vi "Pipe Var Intf - Read Variable - Double.vi"(8 "error in (no error)":errorcluster, 9 "max dims (0: scalar)":i32, 10 "variable name":string, 11 "GOLPI ref. in":T1={"pipe handle"={"lv_proc.dll file path"=path "", "process instance handle"=[], "debug mode"=FALSE, "debug data"=[]}, "fast read timeout [ms]"=500, "fast read settle time [ms]"=10, "fast read to multiple [ms]"=1, "max elements per input line"=100, "slow read timeout [ms]"=5000, "stdin double format specifier"="%_16e", "max elements per stdout output column"=100, "console mode bitstream"=FALSE, "bitstream first read timeout [ms]"=1000, "bitstream read timeout [ms]"=50, "struct transfer possible"=FALSE, "matlab mode"=FALSE, "var pipe write timeout [ms]"=5000, "variable pipe mode"=FALSE, "variable pipe buffer size [Bytes]"=10000000, "variable pipe block size [Bytes]"=1000000} {"variable pipe block size [Bytes]" format="%.0p"; "variable pipe buffer size [Bytes]" format="%.0p"}) -> (0 "error out":errorcluster, 2 "data out":dbl[][](array[numeric]), 3 "GOLPI ref. out":T1={"pipe handle"={"lv_proc.dll file path"=path "", "process instance handle"=[], "debug mode"=FALSE, "debug data"=[]}, "fast read timeout [ms]"=500, "fast read settle time [ms]"=10, "fast read to multiple [ms]"=1, "max elements per input line"=100, "slow read timeout [ms]"=5000, "stdin double format specifier"="", "max elements per stdout output column"=100, "console mode bitstream"=FALSE, "bitstream first read timeout [ms]"=1000, "bitstream read timeout [ms]"=50, "struct transfer possible"=FALSE, "matlab mode"=FALSE, "var pipe write timeout [ms]"=5000, "variable pipe mode"=FALSE, "variable pipe buffer size [Bytes]"=10000000, "variable pipe block size [Bytes]"=1000000} {"variable pipe block size [Bytes]" format="%.0p"; "variable pipe buffer size [Bytes]" format="%.0p"})   [LabVIEW 2020, in "GOLPI library.lvlib"]
doc: "Read matrix from Octave using pipe variable interface. In case of compatible non-doubles, casts to double. max dims defines maximum expected dimensions count."
uses:
  GOLPI library.lvlib
  Public/GOLPI reference Type Def.ctl
  LV Process source distribution/Pipe Handle.ctl
  <vilib>/Utility/error.llb/Error Cluster From Error Code.vi
  <vilib>/ErrorRing/Error Ring.xnode
  LV Process source distribution/LV Process library.lvlib
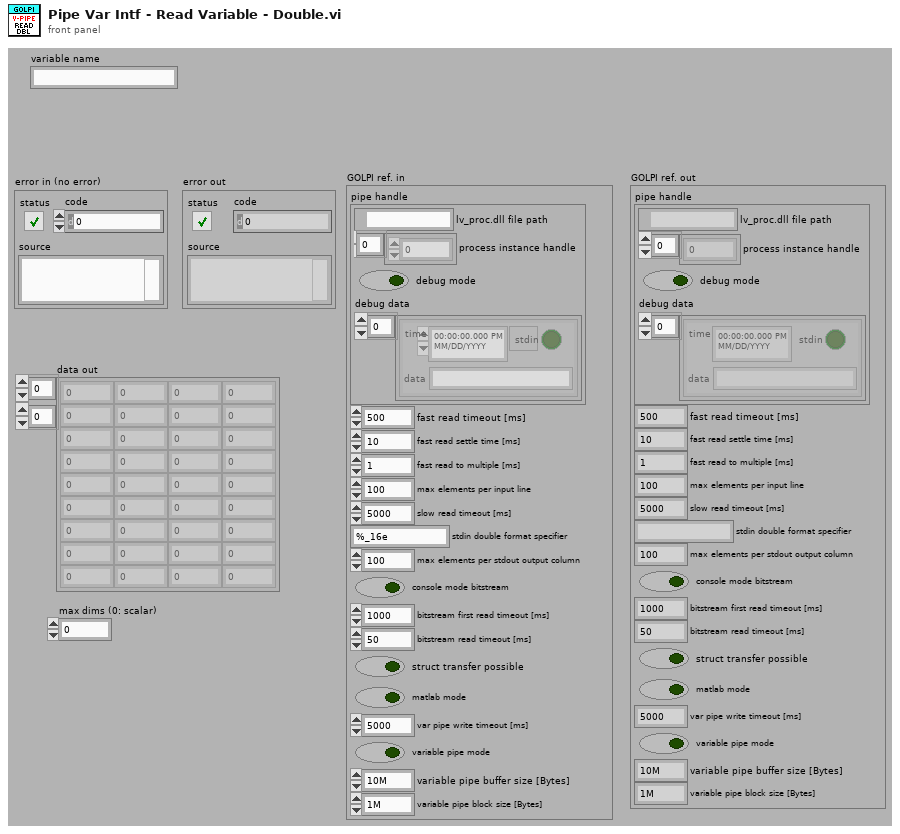
[diagram p1: front panel]
types:
  T1 = typedef "GOLPI library.lvlib/GOLPI reference Type Def.ctl" = cluster{"pipe handle":T2, "fast read timeout [ms]":u32, "fast read settle time [ms]":u32, "fast read to multiple [ms]":u32, "max elements per input line":u32, "slow read timeout [ms]":u32, "stdin double format specifier":string, "max elements per stdout output column":u32, "console mode bitstream":bool, "bitstream first read timeout [ms]":u32, "bitstream read timeout [ms]":u32, "struct transfer possible":bool, "matlab mode":bool, "var pipe write timeout [ms]":u32, "variable pipe mode":bool, "variable pipe buffer size [Bytes]":u32, "variable pipe block size [Bytes]":u32}
  T2 = typedef "LV Process library.lvlib/Pipe Handle.ctl" = cluster{"lv_proc.dll file path":path, "process instance handle":u32[], "debug mode":bool, "debug data":cluster{"time":timestamp, "stdin":bool, "data":string}[]}
  T3 = typedef "GOLPI library.lvlib/Pipe Var Intf - Data Type.ctl" = enum16{"error", "String", "int8", "uint8", "int16", "uint16", "int32", "uint32", "double", "cplx double", "single", "cplx single"}
  T4 = enum16{"big-endian, network order", "native, host order", "little-endian"}
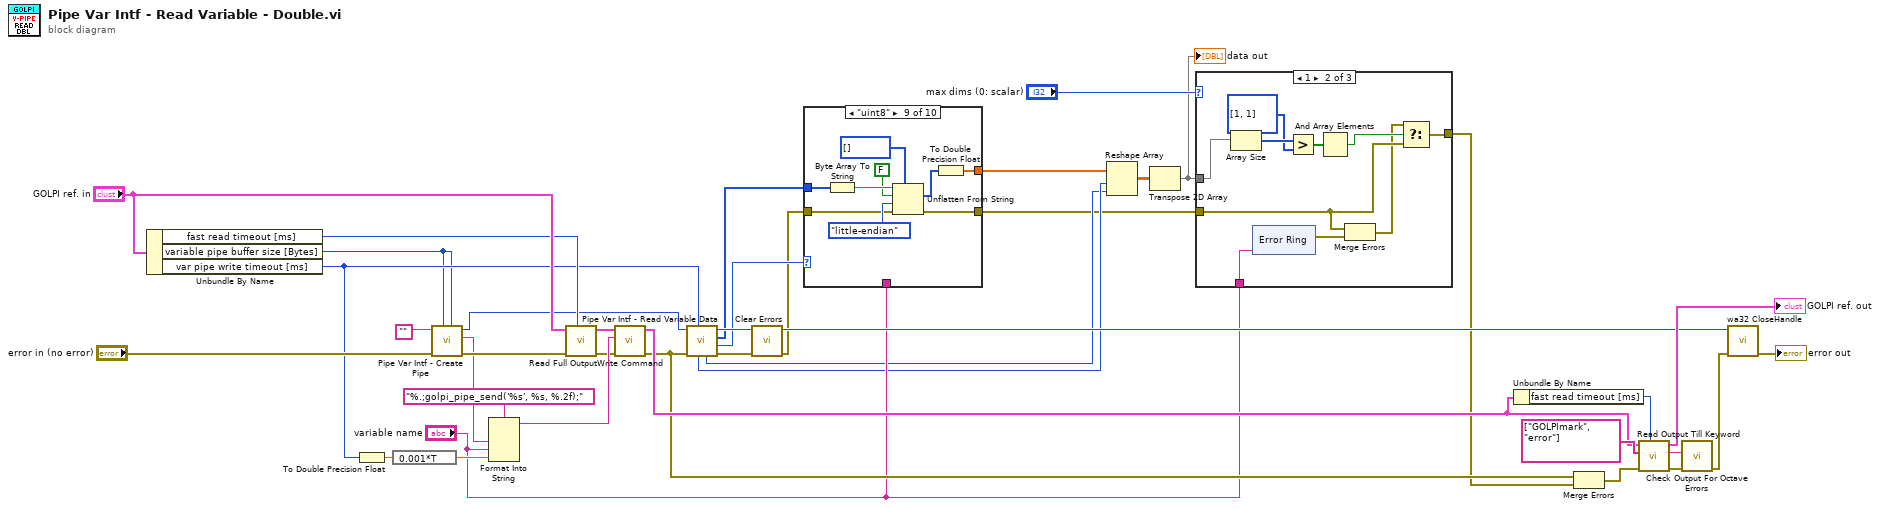
[diagram p0: block diagram]
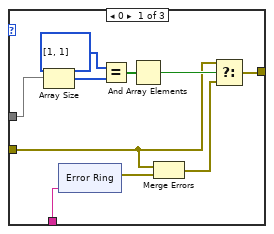
[diagram p2: hidden frame]
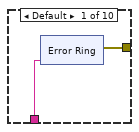
[diagram p4: hidden frame]
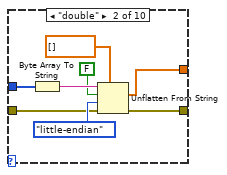
[diagram p5: hidden frame]
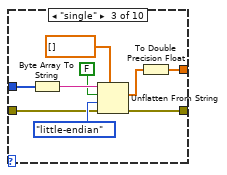
[diagram p6: hidden frame]
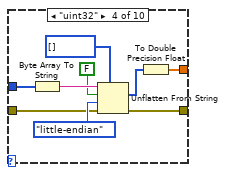
[diagram p7: hidden frame]
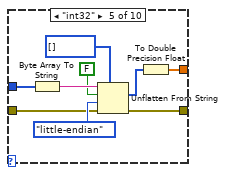
[diagram p8: hidden frame]
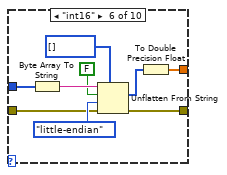
[diagram p9: hidden frame]
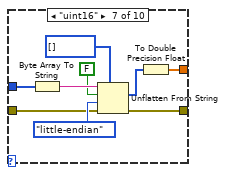
[diagram p10: hidden frame]
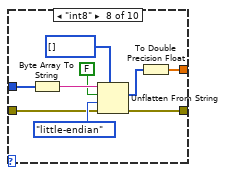
[diagram p11: hidden frame]
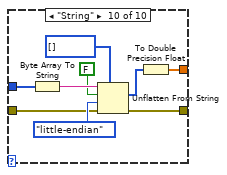
[diagram p12: hidden frame]
diagram:
  n1 = Unbundle By Name("GOLPI ref. in") -> ("fast read timeout [ms]"=w22:u32, "variable pipe buffer size [Bytes]"=w3:u32, "var pipe write timeout [ms]"=w17:u32)
  n2 = To Double Precision Float(number=w17) -> (double precision float=w35:dbl)
  n3 = expression code="0.001*T"(w35) -> (w36:dbl)
  n4 = call "Pipe Var Intf - Create Pipe.vi"("outBufferSize (256k)"=w3, "inBufferSize (256k)"=w3, "error in (no error)"="error in (no error)", "pipe name in (leave empty to generate random name)"="") -> ("error out"=w25:errorcluster, "pipe name out"=w19:string, "pipe handle out"=w18:i32)  [unwired: 5 in]
  n5 = Format Into String(format string="%.;golpi_pipe_send('%s', %s, %.2f);", w19, "variable name", w36) -> (resulting string=w38:string)  [unwired: 2 in, 1 out]
  n6 = call "Read Full Output.vi"("timeout [ms]"=w22, "error in"=w25, "GOLPI ref. in"="GOLPI ref. in") -> ("error out"=w26:errorcluster, "GOLPI ref. out"=w23:T1)  [unwired: 5 in, 2 out]
  n7 = call "Write Command.vi"("error in"=w26, "command"=w38, "GOLPI ref. in"=w23) -> ("error out"=w14:errorcluster, "GOLPI ref. out"=w27:T1)  [unwired: 7 in]
  n8 = call "Pipe Var Intf - Read Variable Data.vi"("timeout [ms]"=w17, "error in (no error)"=w14, "pipe handle"=w18) -> ("error out"=w16:errorcluster, "data type"=w13:T3, "data out"=w12:u8[], "pipe handle out"=w15:i32, "rows"=w5:i32, "columns"=w6:i32)  [unwired: 3 in]
  n9 = call <vilib>:"Clear Errors.vi"("error in (no error)"=w16) -> ("error out"=w11:errorcluster)  [unwired: 5 in, 1 out]
  n10 = case shown="\"uint8\"" w13 {
    tunnel: w12 -> [_ w52 w61 w70 w79 w88 w97 w106 w115 w124]
    tunnel: w11 -> [_ w51 w60 w69 w78 w87 w96 w105 w114 w123]
    tunnel: [w41 w49 w58 w67 w76 w85 w94 w103 w112 w121] -> w2
    tunnel: "variable name" -> [w40 _ _ _ _ _ _ _ _ _]
    tunnel: [_ w50 w57 w66 w75 w84 w93 w102 w111 w120] -> w7
    frame Default {
      n11 = xnode "Error Ring"("parameter 0"=w40) -> ("error out"=w41:errorcluster)
    }
    frame "double" {
      n12 = Byte Array To String(unsigned byte array=w52) -> (string=w56:string)
      n13 = Unflatten From String(type=dbl[] [], binary string=w56, data includes array or string size? (T)=FALSE, byte order (0:big-endian, network order)=T4."little-endian", error in (no error)=w51) -> (value=w50:dbl[], error out=w49:errorcluster)  [unwired: 1 out]
    }
    frame "single" {
      n14 = Byte Array To String(unsigned byte array=w61) -> (string=w65:string)
      n15 = Unflatten From String(type=sgl[] [], binary string=w65, data includes array or string size? (T)=FALSE, byte order (0:big-endian, network order)=T4."little-endian", error in (no error)=w60) -> (value=w59:sgl[], error out=w58:errorcluster)  [unwired: 1 out]
      n16 = To Double Precision Float(number=w59) -> (double precision float=w57:dbl[])
    }
    frame "uint32" {
      n17 = Byte Array To String(unsigned byte array=w70) -> (string=w74:string)
      n18 = Unflatten From String(type=u32[] [], binary string=w74, data includes array or string size? (T)=FALSE, byte order (0:big-endian, network order)=T4."little-endian", error in (no error)=w69) -> (value=w68:u32[], error out=w67:errorcluster)  [unwired: 1 out]
      n19 = To Double Precision Float(number=w68) -> (double precision float=w66:dbl[])
    }
    frame "int32" {
      n20 = Byte Array To String(unsigned byte array=w79) -> (string=w83:string)
      n21 = Unflatten From String(type=i32[] [], binary string=w83, data includes array or string size? (T)=FALSE, byte order (0:big-endian, network order)=T4."little-endian", error in (no error)=w78) -> (value=w77:i32[], error out=w76:errorcluster)  [unwired: 1 out]
      n22 = To Double Precision Float(number=w77) -> (double precision float=w75:dbl[])
    }
    frame "int16" {
      n23 = Byte Array To String(unsigned byte array=w88) -> (string=w92:string)
      n24 = Unflatten From String(type=i16[] [], binary string=w92, data includes array or string size? (T)=FALSE, byte order (0:big-endian, network order)=T4."little-endian", error in (no error)=w87) -> (value=w86:i16[], error out=w85:errorcluster)  [unwired: 1 out]
      n25 = To Double Precision Float(number=w86) -> (double precision float=w84:dbl[])
    }
    frame "uint16" {
      n26 = Byte Array To String(unsigned byte array=w97) -> (string=w101:string)
      n27 = Unflatten From String(type=u16[] [], binary string=w101, data includes array or string size? (T)=FALSE, byte order (0:big-endian, network order)=T4."little-endian", error in (no error)=w96) -> (value=w95:u16[], error out=w94:errorcluster)  [unwired: 1 out]
      n28 = To Double Precision Float(number=w95) -> (double precision float=w93:dbl[])
    }
    frame "int8" {
      n29 = Byte Array To String(unsigned byte array=w106) -> (string=w110:string)
      n30 = Unflatten From String(type=i8[] [], binary string=w110, data includes array or string size? (T)=FALSE, byte order (0:big-endian, network order)=T4."little-endian", error in (no error)=w105) -> (value=w104:i8[], error out=w103:errorcluster)  [unwired: 1 out]
      n31 = To Double Precision Float(number=w104) -> (double precision float=w102:dbl[])
    }
    frame "uint8" {
      n32 = Byte Array To String(unsigned byte array=w115) -> (string=w119:string)
      n33 = Unflatten From String(type=u8[] [], binary string=w119, data includes array or string size? (T)=FALSE, byte order (0:big-endian, network order)=T4."little-endian", error in (no error)=w114) -> (value=w113:u8[], error out=w112:errorcluster)  [unwired: 1 out]
      n34 = To Double Precision Float(number=w113) -> (double precision float=w111:dbl[])
    }
    frame "String" {
      n35 = Byte Array To String(unsigned byte array=w124) -> (string=w128:string)
      n36 = Unflatten From String(type=u8[] [], binary string=w128, data includes array or string size? (T)=FALSE, byte order (0:big-endian, network order)=T4."little-endian", error in (no error)=w123) -> (value=w122:u8[], error out=w121:errorcluster)  [unwired: 1 out]
      n37 = To Double Precision Float(number=w122) -> (double precision float=w120:dbl[])
    }
  }
  n38 = Reshape Array(w7, w6, w5) -> (w8:dbl[][])
  n39 = Transpose 2D Array(2D array=w8) -> (transposed array=w4:dbl[][])
  "data out" <- w4
  n40 = case shown="1" "max dims (0: scalar)" {
    tunnel: w4 -> [w138 w155 _]
    tunnel: w2 -> [w130 w147 w163]
    tunnel: [w133 w154 w163] -> w1
    tunnel: "variable name" -> [w132 w153 _]
    frame 0 {
      n41 = Array Size(array=w138) -> (size(s)=w137:i32[])
      n42 = xnode "Error Ring"("parameter 0"=w132) -> ("error out"=w131:errorcluster)
      n43 = Equal?(x=i32[] [1, 1], y=w137) -> (x = y?=w135:bool[])
      n44 = And Array Elements(Boolean array=w135) -> (logical AND=w134:bool)
      n45 = Merge Errors(w130, w131) -> (w129:errorcluster)
      n46 = Select(t=w130, s=w134, f=w129) -> (s? t:f=w133:errorcluster)
    }
    frame 1 {
      n47 = Array Size(array=w155) -> (size(s)=w151:i32[])
      n48 = xnode "Error Ring"("parameter 0"=w153) -> ("error out"=w152:errorcluster)
      n49 = Greater?(x=w151, y=i32[] [1, 1] ("x")) -> (0:w149:bool[])
      n50 = And Array Elements(Boolean array=w149) -> (logical AND=w148:bool)
      n51 = Merge Errors(w147, w152) -> (w146:errorcluster)
      n52 = Select(t=w146, s=w148, f=w147) -> (s? t:f=w154:errorcluster)
    }
    frame Default {
    }
  }
  n53 = Unbundle By Name(w27) -> ("fast read timeout [ms]"=w33:u32)
  n54 = Merge Errors(w14, w1) -> (w21:errorcluster)
  n55 = call "Read Output Till Keyword.vi"("timeout [ms]"=w33, "error in"=w21, "keywords"=string[] ["GOLPImark", "error"], "GOLPI ref. in"=w27) -> ("error out"=w32:errorcluster, "read buffer"=w31:string, "GOLPI ref. out"=→"GOLPI ref. out":T1)  [unwired: 4 in, 1 out]
  n56 = call "Check Output For Octave Errors.vi"("error in"=w32, "read buffer"=w31) -> ("error out"=w28:errorcluster)  [unwired: 9 in]
  n57 = call "wa32 CloseHandle.vi"("error in"=w28, "handle"=w15) -> ("error out"=→"error out":errorcluster)  [unwired: 9 in]
